vi "rs3 wait for frames4.vi"(8 "error in (no error)":errorcluster, 10 "timeout (ms)":u64, 11 "device in":u64) -> (0 "error out":errorcluster, 3 "device out":u64)   [LabVIEW 2023]
doc: "Block until new frames are available. Returns the next FRAME handle when available."
uses:
  realsense2.dll
panel:
  # "RS3 Wait for Frames"
  # "(C) Intel Corp. 2017,  AGJ"
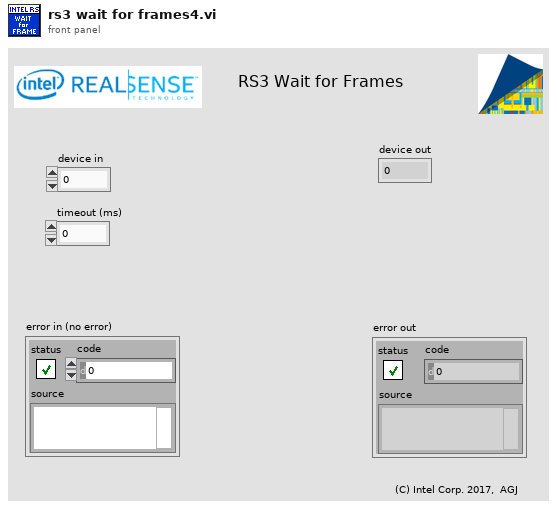
[diagram p1: front panel]
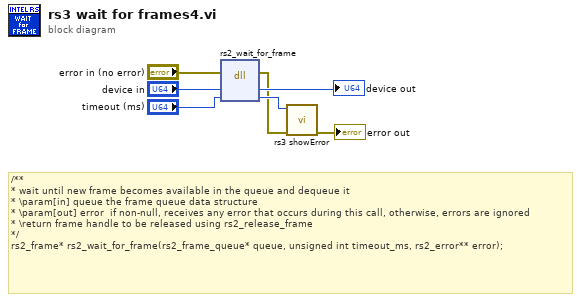
[diagram p0: block diagram]
diagram:
  # "/**\n* wait until new frame becomes available in the queue and dequeue it\n* \\param[in] queue the frame queue data structure\n* \\param[out] error  if non-null, receives any error that occurs during this call, otherwise, errors are ignored\n* \\return frame handle to be released using rs2_release_frame\n*/\nrs2_frame* rs2_wait_for_frame(rs2_frame_queue* queue, unsigned int timeout_ms, rs2_error** error);"
  n1 = dll-call lib="C:/STEAMSyndicate/RealSenseWrappers/VI Wrappers (add ons) Public/RealSense/realsense2.dll" fn="rs2_wait_for_frame"(error in="error in (no error)", "device"="device in", "error"="timeout (ms)") -> (error out=w3:errorcluster, "device"=→"device out":u64, "error"=w4:u64)  [unwired: 3 in, 1 out]
  n2 = call "rs3 showError.vi"("error in (no error)"=w3, "error"=w4) -> ("error out"=→"error out":errorcluster)  [unwired: 5 in, 4 out]
